vi "removeFormatting.vi"(8 "error in (no error)":errorcluster, 10 "input":string, 11 "PrettyPrinting in":refnum<class "PrettyPrinting.lvclass">) -> (0 "error out":errorcluster, 2 "output":string, 3 "PrettyPrinting out":refnum<class "PrettyPrinting.lvclass">)   [LabVIEW 2011, in "Views.lvlib" / "ViewerTools.lvlib" / "PrettyPrinting.lvclass"]
uses:
  PrettyPrinting.lvclass
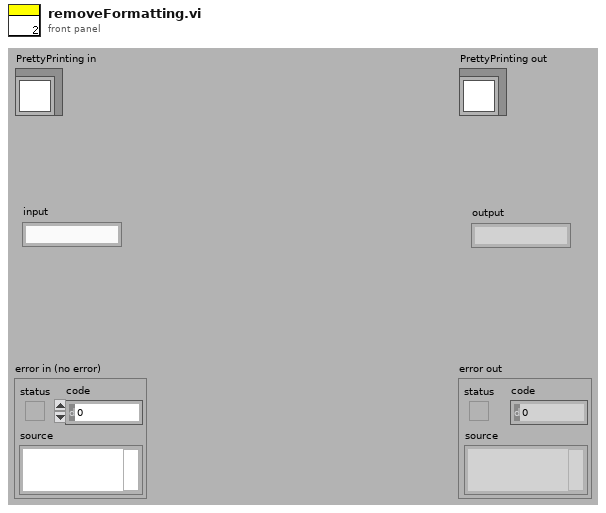
[diagram p1: front panel]
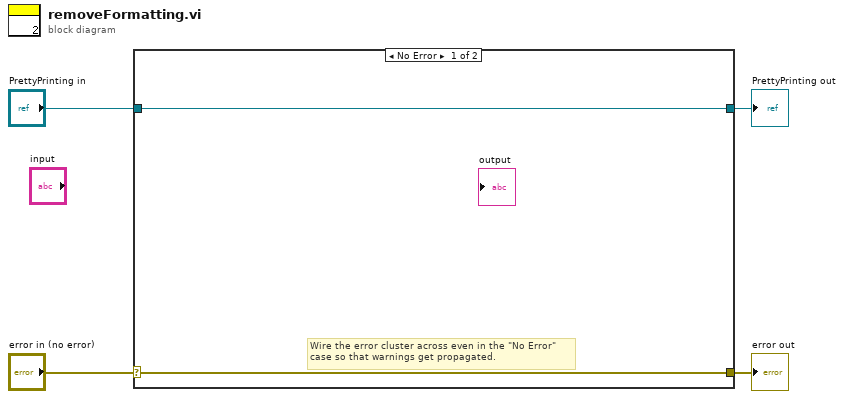
[diagram p0: block diagram]
diagram:
  n1 = case shown="No Error" "error in (no error)" {
    selector: "error in (no error)" -> [w5 w8]
    tunnel: [w5 w8] -> w3
    tunnel: [w6 w7] -> w1
    tunnel: "PrettyPrinting in" -> [w6 w7]
    frame No Error {
      # "Wire the error cluster across even in the \"No Error\"\ncase so that warnings get propagated."
    }
    frame Error {
    }
  }
  "error out" <- w3
  "PrettyPrinting out" <- w1
